vi "Thermocouple Main.vi"() -> ()   [LabVIEW 2020]
doc: "This VI can be used as a launcher VI for the main application or as a debugging tool.\n_____\nBased on Delacor QMH Project Template 5.0.0.82."
uses:
  Libraries/CML UI/MainUI.lvlib
  Libraries/Launcher Support/Launcher Support.lvlib
panel:
  out "Command Line Arguments":string[](array[string])
  out "Module Running?":bool
  out "Status":string
  out "error out":errorcluster
  in  "Stop Module":bool
  in  "Start Module":bool
  # "See the Build_Final_EXE bookmarks on the diagram for instructions on using this VI as a launcher for an EXE."
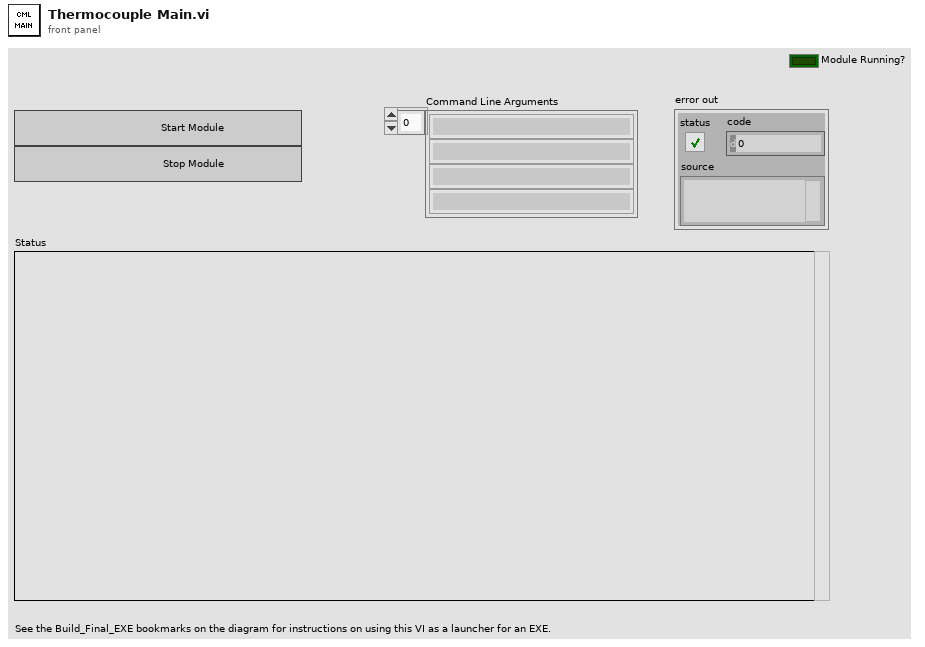
[diagram p1: front panel]
types:
  T1 = enum32{"invalid app kind", "Development System", "Run Time System", "Student Edition", "Embedded LabVIEW", "Evaluation", "Custom"}
  T2 = typedef "MainUI.lvlib/Broadcast Events--cluster.ctl" = cluster{"Module Did Init":refnum<user-event>, "Status Updated":refnum<user-event>, "Error Reported":refnum<user-event>, "Module Did Stop":refnum<user-event>, "Update Module Execution Status":refnum<user-event>}
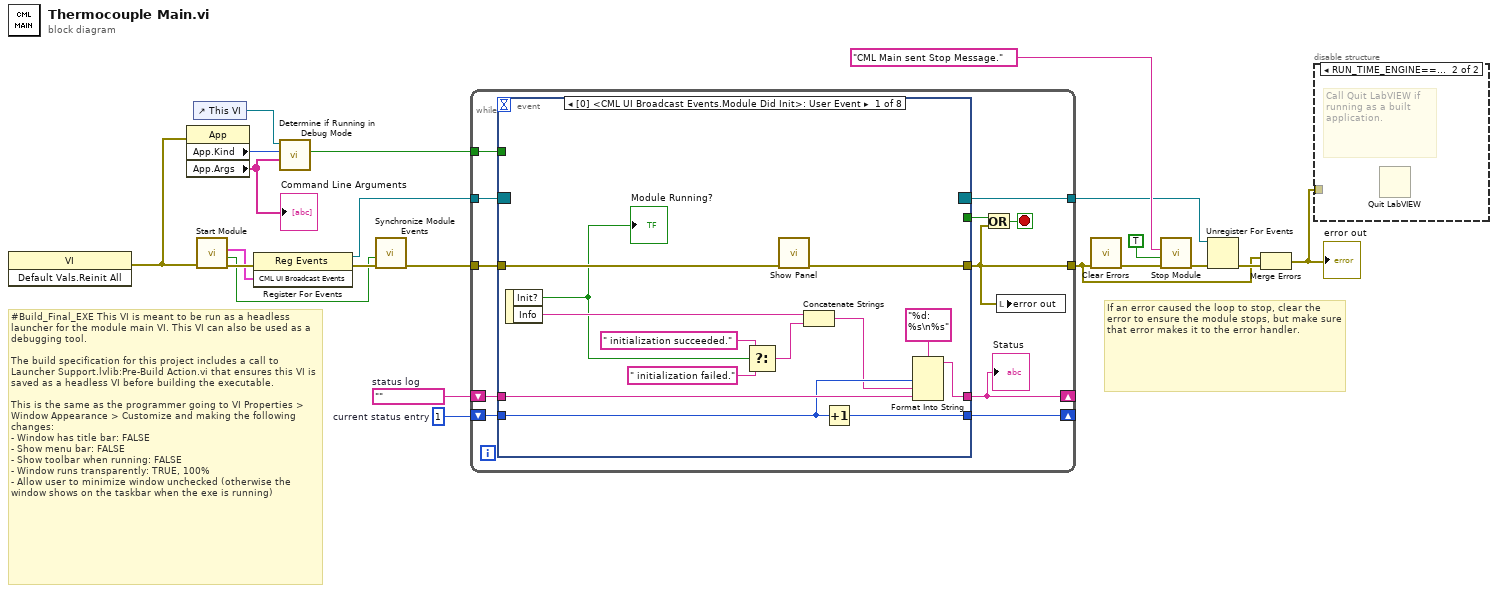
[diagram p0: block diagram]
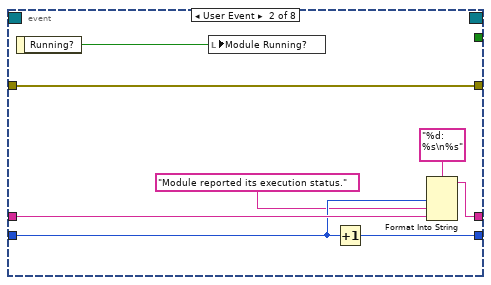
[diagram p2: hidden frame]
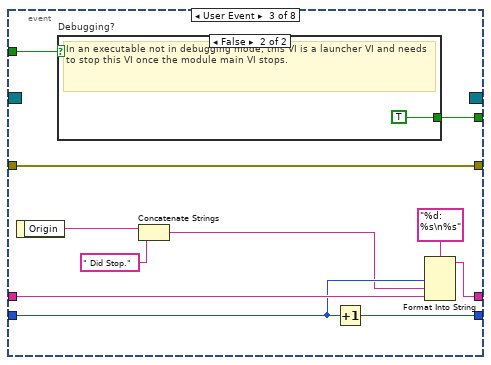
[diagram p3: hidden frame]
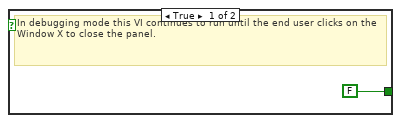
[diagram p4: hidden frame]
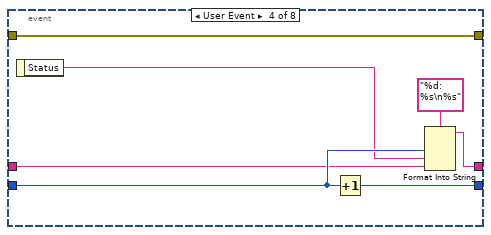
[diagram p5: hidden frame]
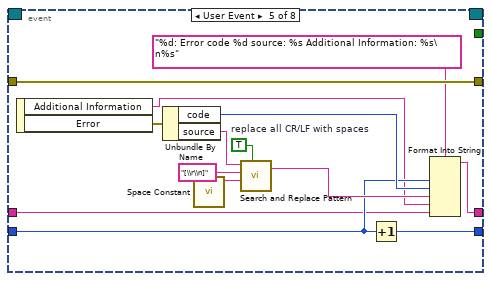
[diagram p6: hidden frame]
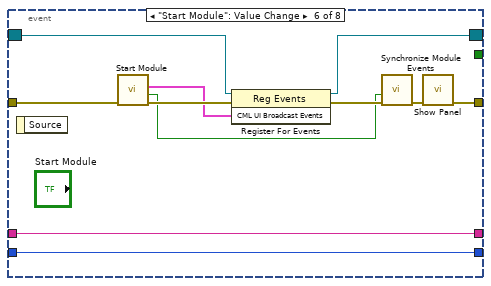
[diagram p7: hidden frame]
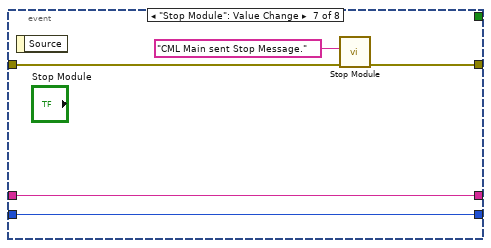
[diagram p8: hidden frame]
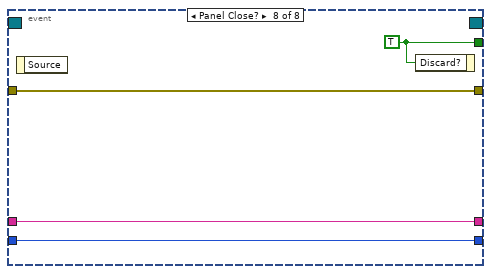
[diagram p9: hidden frame]
diagram:
  w17 = 1  # current status entry
  w18 = ""  # status log
  # "#Build_Final_EXE This VI is meant to be run as a headless launcher for the module main VI. This VI can also be used as a debugging tool. \n\nThe build specification for this project includes a call to Launcher Support.lvlib:Pre-Build Action.vi that ensures this VI is saved as a headless VI before building the executable.\n\nThis is the same as the programmer going to VI Properties > Window Appearance > Customize and making the following changes:\n- Window has title bar: FALSE\n- Show menu bar: FALSE\n- Show toolbar when running: FALSE\n- Window runs transparently: TRUE, 100%\n- Allow user to minimize window unchecked (otherwise the window shows on the taskbar when the exe is running)"
  # "If an error caused the loop to stop, clear the error to ensure the module stops, but make sure that error makes it to the error handler."
  n1 = invoke on="Invoke Node" class="VI" method="Default Vals.Reinit All"() -> (error out=w5:errorcluster)  [unwired: 3 in, 2 out]
  n2 = property on="Property Node" class="App"(error in=w5) -> ("App.Kind"=w1:T1, "App.Args"=w4:string[])  [unwired: 1 in, 2 out]
  "Command Line Arguments" <- w4
  n3 = control-ref of="This VI"() -> (w3:refnum<vi>)
  n4 = call "Start Module.vi"("error in (no error)"=w5) -> ("error out"=w12:errorcluster, "Wait for Event Sync?"=w11:bool, "CML UI Broadcast Events"=w10:T2)  [unwired: 7 in, 1 out]
  n5 = register-events(error in=w12, w10) -> (reference out=w9:refnum<event-registration>, error out=w13:errorcluster)  [unwired: 1 in]
  n6 = call "Determine if Running in Debug Mode.vi"("App.Args"=w4, "App.Kind"=w1, "Launcher VI ref"=w3) -> ("Debug mode?"=w2:bool)  [unwired: 8 in]
  n7 = call "Synchronize Module Events.vi"("error in (no error)"=w13, "Wait for Event Sync?"=w11) -> ("error out"=w7:errorcluster)  [unwired: 9 in]
  n8 = while {
    tunnel: w9 -> [w32]
    tunnel: [w23] -> w6
    shift-right: [w24] -> _
    shift-left: w18 -> [w29]
    shift-right: [w28] -> _
    shift-left: w17 -> [w30]
    tunnel: w7 -> [w26]
    tunnel: [w25] -> w16
    tunnel: w2 -> [w22]
    stop <- w27 stop-if-true
    n9 = event shown="[0] <CML UI Broadcast Events.Module Did Init>: User Event" {
      selector: w32 -> [_ _ _ _ _ w92 _ _]
      dyn-events: [_ _ _ _ _ w91 _ _] -> w25
      timeout: _ -> [_ _ _ _ _ _ _ _]
      tunnel: [_ _ w55 _ _ _ _ w107] -> w31
      tunnel: [w33 w47 w56 w67 w87 w88 w101 w104] -> w23
      tunnel: w30 -> [w42 w51 w62 w70 w77 w95 w102 w105]
      tunnel: w29 -> [w43 w52 w63 w69 w75 w96 w103 w106]
      tunnel: [w40 w49 w60 w71 w78 w96 w103 w106] -> w24
      tunnel: [w41 w50 w61 w73 w76 w95 w102 w105] -> w28
      tunnel: w26 -> [w45 w47 w56 w67 w87 w90 w99 w104]
      tunnel: w22 -> [_ _ w54 _ _ _ _ _]
      event User Event {
        n10 = event-data() -> ("Init?"=w37:bool, "Info"=w39:string)  [unwired: 1 in]
        "Module Running?" <- w37
        n11 = Select(t=" initialization succeeded.", s=w37, f=" initialization failed.") -> (s? t:f=w34:string)
        n12 = call "Show Panel.vi"("error in (no error)"=w45) -> ("error out"=w33:errorcluster)  [unwired: 10 in]
        n13 = Concatenate Strings(w39, w34) -> (w38:string)
        n14 = Increment(x=w42) -> (x+1=w41:i32)
        n15 = Format Into String(format string="%d: %s\n%s", w42, w38, w43) -> (resulting string=w40:string)  [unwired: 2 in, 1 out]
      }
      event User Event {
        n16 = event-data() -> ("Running?"=w46:bool)  [unwired: 1 in]
        n17 = local write "Module Running?"(w46) -> ()
        n18 = Increment(x=w51) -> (x+1=w50:i32)
        n19 = Format Into String(format string="%d: %s\n%s", w51, "Module reported its execution status.", w52) -> (resulting string=w49:string)  [unwired: 2 in, 1 out]
      }
      event User Event {
        n20 = event-data() -> ("Origin"=w59:string)  [unwired: 1 in]
        n21 = case "Debugging?" shown="False" w54 {
          tunnel: [FALSE ("Discard?") TRUE ("Discard?")] -> w55
          frame True {
            # "In debugging mode this VI continues to run until the end user clicks on the Window X to close the panel."
          }
          frame False {
            # "In an executable not in debugging mode, this VI is a launcher VI and needs to stop this VI once the module main VI stops."
          }
        }
        n22 = Concatenate Strings(w59, " Did Stop.") -> (w58:string)
        n23 = Increment(x=w62) -> (x+1=w61:i32)
        n24 = Format Into String(format string="%d: %s\n%s", w62, w58, w63) -> (resulting string=w60:string)  [unwired: 2 in, 1 out]
      }
      event User Event {
        n25 = event-data() -> ("Status"=w68:string)  [unwired: 1 in]
        n26 = Increment(x=w70) -> (x+1=w73:i32)
        n27 = Format Into String(format string="%d: %s\n%s", w70, w68, w69) -> (resulting string=w71:string)  [unwired: 2 in, 1 out]
      }
      event User Event {
        w83 = TRUE  # replace all CR/LF with spaces
        n28 = event-data() -> ("Additional Information"=w74:string, "Error"=w79:errorcluster)  [unwired: 1 in]
        n29 = Unbundle By Name(w79) -> ("code"=w80:i32, "source"=w81:string)
        n30 = call <vilib>:"Space Constant.vi"() -> ("String"=w84:string)
        n31 = call <vilib>:"Search and Replace Pattern.vi"("string"=w81, "regular expression (\"\")"="[\\r\\n]" ("regular expression (\"\")"), "replace string (\"\")"=w84, "replace all? (F)"=w83) -> ("result string"=w82:string)  [unwired: 1 in, 1 out]
        n32 = Increment(x=w77) -> (x+1=w76:i32)
        n33 = Format Into String(format string="%d: Error code %d source: %s Additional Information: %s\n%s", w77, w80, w82, w74, w75) -> (resulting string=w78:string)  [unwired: 2 in, 1 out]
      }
      event "Start Module": Value Change {
        n34 = event-data() -> ()  [unwired: 1 in, 1 out]
        n35 = call "Start Module.vi"("error in (no error)"=w90) -> ("error out"=w97:errorcluster, "Wait for Event Sync?"=w94:bool, "CML UI Broadcast Events"=w93:T2)  [unwired: 7 in, 1 out]
        n36 = register-events(reference=w92, error in=w97, w93) -> (reference out=w91:refnum<event-registration>, error out=w98:errorcluster)
        n37 = call "Synchronize Module Events.vi"("error in (no error)"=w98, "Wait for Event Sync?"=w94) -> ("error out"=w89:errorcluster)  [unwired: 9 in]
        n38 = call "Show Panel.vi"("error in (no error)"=w89) -> ("error out"=w88:errorcluster)  [unwired: 10 in]
      }
      event "Stop Module": Value Change {
        n39 = event-data() -> ()  [unwired: 1 in, 1 out]
        n40 = call "Stop Module.vi"("error in (no error)"=w99, "Origin"="CML Main sent Stop Message.") -> ("error out"=w101:errorcluster)  [unwired: 9 in]
      }
      event Panel Close? {
        w107 = TRUE ("Discard?")
        n41 = event-data() -> ()  [unwired: 1 in, 1 out]
        n42 = event-data ("Event Filter Node")("Discard?"=w107) -> ()  [unwired: 1 in, 1 out]
      }
    }
    "Status" <- w24
    n43 = Or(x=w31, y=w23) -> (x .or. y?=w27:bool)
    n44 = local write "error out"(w23) -> ()
  }
  n45 = call <vilib>:"Clear Errors.vi"("error in (no error)"=w6) -> ("error out"=w14:errorcluster)  [unwired: 5 in, 1 out]
  n46 = call "Stop Module.vi"("error in (no error)"=w14, "Wait for Module to Stop? (F)"=TRUE ("Wait for Module to stop?"), "Origin"="CML Main sent Stop Message.") -> ("error out"=w20:errorcluster)  [unwired: 8 in]
  n47 = Unregister For Events(event registration refnum=w16, error in=w20) -> (error out=w21:errorcluster)
  n48 = Merge Errors(w6, w21) -> (w8:errorcluster)
  "error out" <- w8
  n49 = disable-structure "Conditional Disable Structure" shown="RUN_TIME_ENGINE==True" {
    disable-tunnel: w8 -> [_ _]
    frame condition #0 (active) {
    }
    frame condition #1 {
      # "Call Quit LabVIEW if running as a built application."
      n50 = Quit LabVIEW() -> ()  [unwired: 1 in]
    }
  }
